vi "calc unit vector comp start.vi"(9 "event data at origin in":T1={"position [km]"=0.0, "time [nsec]"=20}, 10 "event data along axis in":T1={"position [km]"=384400.0, "time [nsec]"=365}, 11 "speed of light [m/s]":sgl=300000000.0) -> (3 "component of unit vector":sgl=-0.26925078)   [LabVIEW 2014]
doc: "Calc Unit Vector\n\nEngenders the component of the unit vector along the given axis of a source based off of the following inputs: speed of light, position at sensor and origin [km] , and time at sensor and origin [nsec].\n\nCalculations:\n\ndta (time interval from orgin to sensor) [sec] = time at sensor [nsec] - time at origin [nsec] \n\ndpa (position of sensor along axis) [m] = position at sensor [km] - position at origin [km] \n\ncomponent of unit vector of a source = -(speed of light * dta) / dpa\n\nBeverly Abadines\nPHY 350: E2"
uses:
  typedefs/event cluster typedef.ctl
panel:
  # "needs work in BD, and make into a fully funtional subvi\n\nsee BD for algorithm"
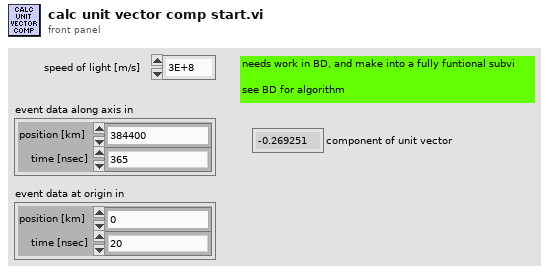
[diagram p1: front panel]
types:
  T1 = typedef "event cluster typedef.ctl" = cluster{"position [km]":sgl, "time [nsec]":i64}
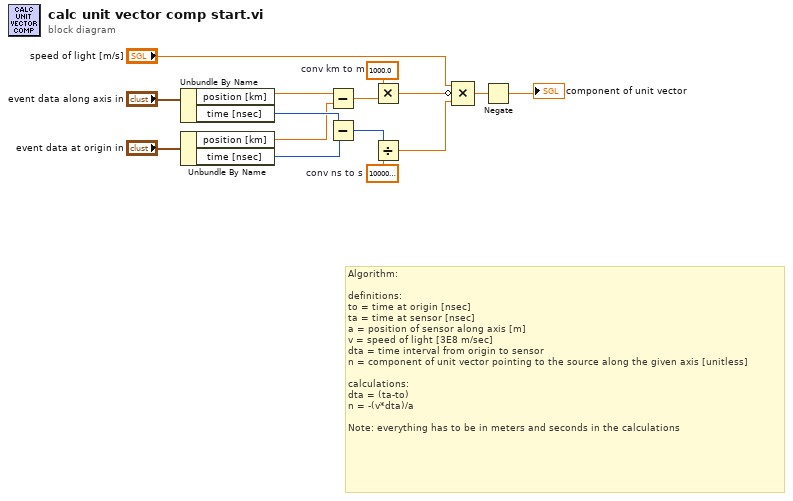
[diagram p0: block diagram]
diagram:
  w6 = sgl 1000.0  # conv km to m
  w10 = sgl 1000000000.0  # conv ns to s
  # "Algorithm:\n\ndefinitions:\nto = time at origin [nsec]\nta = time at sensor [nsec]\na = position of sensor along axis [m]\nv = speed of light [3E8 m/sec]\ndta = time interval from origin to sensor\nn = component of unit vector pointing to the source along the given axis [unitless]\n\ncalculations:\ndta = (ta-to)\nn = -(v*dta)/a\n\nNote: everything has to be in meters and seconds in the calculations"
  n1 = Unbundle By Name("event data along axis in") -> ("position [km]"=w8:sgl, "time [nsec]"=w13:i64)
  n2 = Unbundle By Name("event data at origin in") -> ("position [km]"=w9:sgl, "time [nsec]"=w12:i64)
  n3 = Subtract(x=w8, y=w9) -> (x-y=w7:sgl)
  n4 = Subtract(x=w13, y=w12) -> (x-y=w11:i64)
  n5 = Multiply(x=w6, y=w7) -> (x*y=w4:sgl)
  n6 = Divide(x=w11, y=w10) -> (x/y=w3:sgl)
  n7 = Compound Arithmetic op=MULTIPLY("speed of light [m/s]", invert w4, w3) -> (w2:sgl)
  n8 = Negate(x=w2) -> (-x=→"component of unit vector":sgl)
